vi "MSScript_SubVI_ParamName&Val.vi"(2 "PARAMs":cluster{"Str":string, "Start":i32}[](array[cluster])) -> (5 "PARAM.NAMEs":cluster{"Str":string, "Start":i32}[](array[cluster]), 6 "PARAM.VALs":cluster{"Str":string, "Start":i32}[](array[cluster]), 7 "PARAM.EqualSign":cluster{"Str":string, "Start":i32}[](array[cluster]), 8 "Equal sign no found":bool[](array[boolean]))   [LabVIEW 2018, in "MSScript.lvclass"]
uses:
  MSScript.lvclass
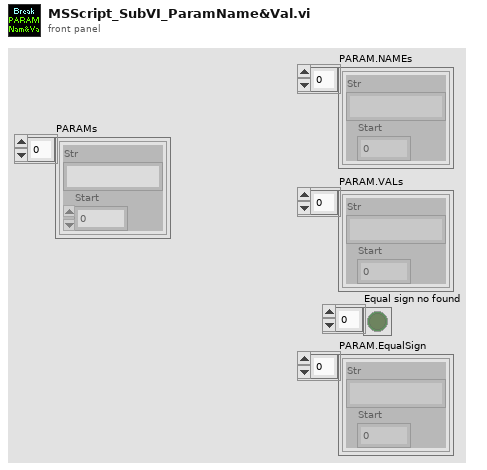
[diagram p1: front panel]
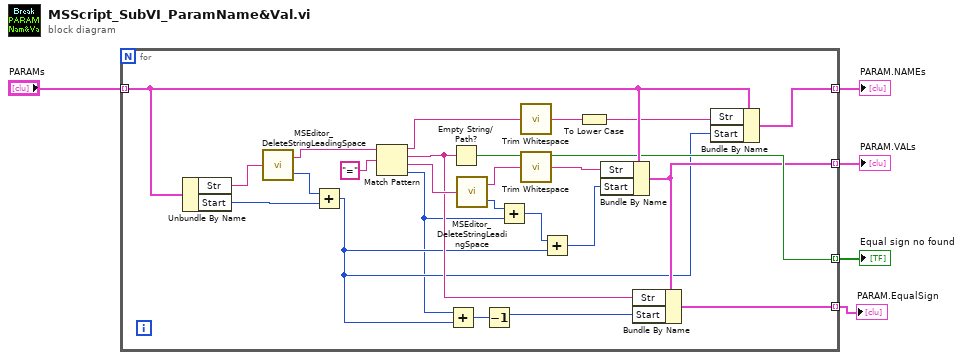
[diagram p0: block diagram]
diagram:
  n1 = for {
    tunnel: "PARAMs" -> [w18] mode=indexing
    tunnel: [w16] -> w4 mode=indexing
    tunnel: [w14] -> w3 mode=indexing
    tunnel: [w15] -> w2 mode=indexing
    tunnel: [w11] -> w1 mode=indexing
    n2 = Unbundle By Name(w18) -> ("Str"=w29:string, "Start"=w27:i32)
    n3 = call "MSEditor_DeleteStringLeadingSpace.vi"("string in"=w29) -> ("string after leading space"=w25:string, "offset past leading space"=w28:i32)
    n4 = Add(x=w28, y=w27) -> (x+y=w7:i32)
    n5 = Match Pattern(string=w25, regular expression="=") -> (before substring=w17:string, match substring=w12:string, after substring=w24:string, offset past match=w6:i32)  [unwired: 1 in]
    n6 = Add(x=w6, y=w7) -> (x+y=w8:i32)
    n7 = Empty String/Path?(string/path=w12) -> (empty?=w15:bool)
    n8 = call "MSEditor_DeleteStringLeadingSpace.vi"("string in"=w24) -> ("string after leading space"=w21:string, "offset past leading space"=w23:i32)
    n9 = Decrement(x=w8) -> (x-1=w13:i32)
    n10 = Add(x=w23, y=w6) -> (x+y=w22:i32)
    n11 = call <vilib>:"Trim Whitespace.vi"("string"=w17) -> ("trimmed string"=w10:string)  [unwired: 1 in]
    n12 = call <vilib>:"Trim Whitespace.vi"("string"=w21) -> ("trimmed string"=w20:string)  [unwired: 1 in]
    n13 = Add(x=w22, y=w7) -> (x+y=w19:i32)
    n14 = To Lower Case(string=w10) -> (all lower case string=w9:string)
    n15 = Bundle By Name(cluster=w18, "Str"=w20, "Start"=w19) -> (w14:cluster{"Str":string, "Start":i32})
    n16 = Bundle By Name(cluster=w14, "Str"=w12, "Start"=w13) -> (w11:cluster{"Str":string, "Start":i32})
    n17 = Bundle By Name(cluster=w18, "Str"=w9, "Start"=w7) -> (w16:cluster{"Str":string, "Start":i32})
  }
  "PARAM.NAMEs" <- w4
  "PARAM.VALs" <- w3
  "Equal sign no found" <- w2
  "PARAM.EqualSign" <- w1
